vi "Crosshairs.vi"(1 "Potent":dbl) -> ()   [LabVIEW 2012]
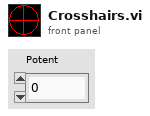
[diagram p1: front panel]
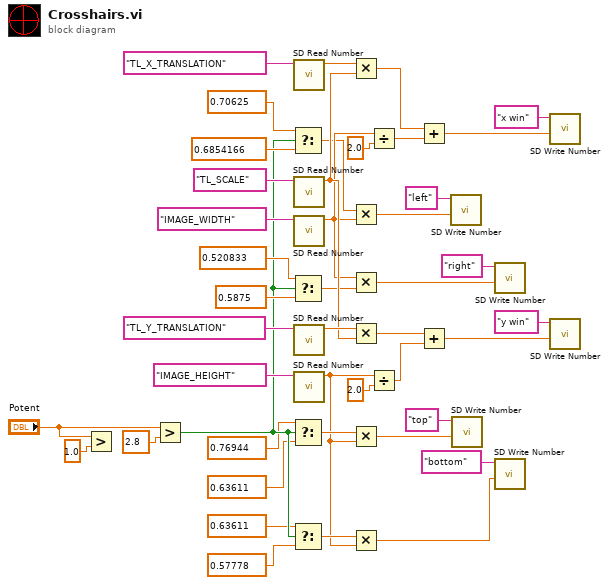
[diagram p0: block diagram]
diagram:
  n1 = Greater?(x="Potent", y=1.0) -> ()  [unwired: 1 out]
  n2 = Greater?(x="Potent", y=2.8) -> (0:w10:bool)
  n3 = Select(t=0.70625, s=w10, f=0.6854166) -> (s? t:f=w14:dbl)
  n4 = Select(t=0.520833, s=w10, f=0.5875) -> (s? t:f=w17:dbl)
  n5 = Select(t=0.76944, s=w10, f=0.63611) -> (s? t:f=w7:dbl)
  n6 = Select(t=0.63611, s=w10, f=0.57778) -> (s? t:f=w6:dbl)
  n7 = call <vilib>:"SD Read Number.vi"("Name"="TL_X_TRANSLATION") -> ("Numeric"=w33:dbl)  [unwired: 8 in, 2 out]
  n8 = call <vilib>:"SD Read Number.vi"("Name"="TL_SCALE") -> ("Numeric"=w36:dbl)  [unwired: 8 in, 2 out]
  n9 = call <vilib>:"SD Read Number.vi"("Name"="IMAGE_WIDTH") -> ("Numeric"=w15:dbl)  [unwired: 8 in, 2 out]
  n10 = call <vilib>:"SD Read Number.vi"("Name"="TL_Y_TRANSLATION") -> ("Numeric"=w38:dbl)  [unwired: 8 in, 2 out]
  n11 = call <vilib>:"SD Read Number.vi"("Name"="IMAGE_HEIGHT") -> ("Numeric"=w3:dbl)  [unwired: 8 in, 2 out]
  n12 = Multiply(x=w33, y=w36) -> (x*y=w29:dbl)
  n13 = Multiply(x=w14, y=w15) -> (x*y=w13:dbl)
  n14 = Multiply(x=w15, y=w17) -> (x*y=w16:dbl)
  n15 = Multiply(x=w38, y=w36) -> (x*y=w37:dbl)
  n16 = Multiply(x=w7, y=w3) -> (x*y=w2:dbl)
  n17 = Multiply(x=w6, y=w3) -> (x*y=w1:dbl)
  n18 = Divide(x=w15, y=2.0) -> (x/y=w28:dbl)
  n19 = Divide(x=w3, y=2.0) -> (x/y=w30:dbl)
  n20 = Add(x=w29, y=w28) -> (x+y=w27:dbl)
  n21 = Add(x=w37, y=w30) -> (x+y=w42:dbl)
  n22 = call <vilib>:"SD Write Number.vi"("Numeric"=w13, "Name"="left") -> ()  [unwired: 8 in, 2 out]
  n23 = call <vilib>:"SD Write Number.vi"("Numeric"=w2, "Name"="top") -> ()  [unwired: 8 in, 2 out]
  n24 = call <vilib>:"SD Write Number.vi"("Numeric"=w16, "Name"="right") -> ()  [unwired: 8 in, 2 out]
  n25 = call <vilib>:"SD Write Number.vi"("Numeric"=w1, "Name"="bottom") -> ()  [unwired: 8 in, 2 out]
  n26 = call <vilib>:"SD Write Number.vi"("Numeric"=w27, "Name"="x win") -> ()  [unwired: 8 in, 2 out]
  n27 = call <vilib>:"SD Write Number.vi"("Numeric"=w42, "Name"="y win") -> ()  [unwired: 8 in, 2 out]
